vi "ChParamGetRef.vi"(0 "Ch Received in":refnum<vi>, 1 "Channel OFF delay":refnum<vi>, 2 "Channel On Delay in":refnum<vi>, 3 "Number Of Retry in":refnum<vi>, 4 "SW Retry Delay":refnum<vi>, 5 "Retry Delay in":refnum<vi>, 6 "Active on startup":refnum<vi>, 7 "SW Number Of Retry":refnum<vi>, 8 "Reset Status Delay":refnum<vi>, 9 "I/O control":refnum<vi>, 10 "Init":bool, 11 "Current Threshold in":refnum<vi>, 12 "Ch General data":refnum<vi>, 13 "Comm. control":refnum<vi>) -> (14 "Reset Status Delay out":refnum<vi>, 16 "Channel On Delay out":refnum<vi>, 17 "Ch General data out":refnum<vi>, 18 "Channel OFF delay out":refnum<vi>, 19 "Comm. control out":refnum<vi>, 20 "Ch Received out":refnum<vi>, 21 "SW Retry Delay out":refnum<vi>, 22 "Current Threshold  out":refnum<vi>, 23 "Active on startup out":refnum<vi>, 24 "SW Number Of Retry out":refnum<vi>, 25 "Retry Delay out":refnum<vi>, 26 "Number Of Retry out":refnum<vi>, 27 "I/O control out":refnum<vi>)   [LabVIEW 2017]
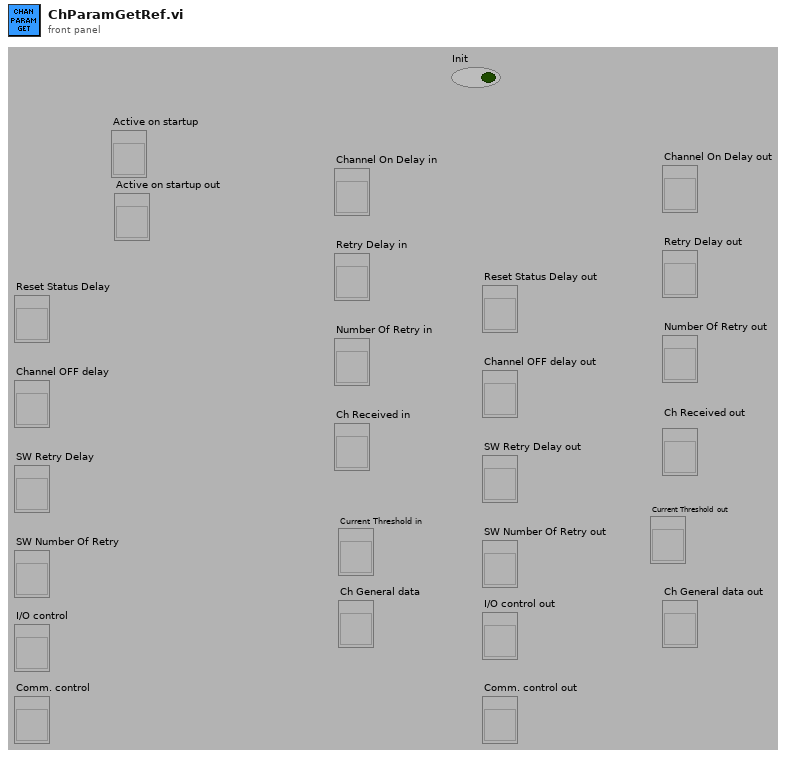
[diagram p1: front panel]
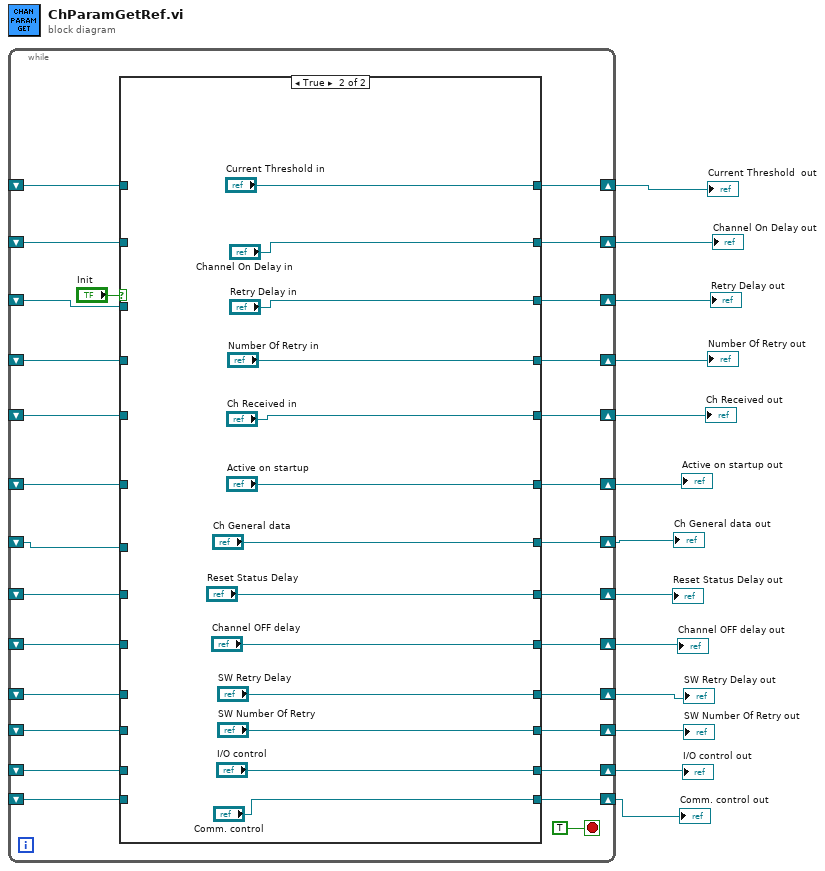
[diagram p0: block diagram]
diagram:
  n1 = while {
    shift-right: [w30] -> w9
    shift-left: _ -> [w36]
    shift-right: [w40] -> w13
    shift-left: _ -> [w35]
    shift-right: [w39] -> w12
    shift-left: _ -> [w34]
    shift-right: [w38] -> w11
    shift-left: _ -> [w33]
    shift-right: [w37] -> w10
    shift-left: _ -> [w32]
    shift-right: [w29] -> w8
    shift-left: _ -> [w28]
    shift-right: [w27] -> w7
    shift-left: _ -> [w26]
    shift-right: [w25] -> w5
    shift-left: _ -> [w19]
    shift-right: [w24] -> w6
    shift-left: _ -> [w18]
    shift-right: [w23] -> w4
    shift-left: _ -> [w17]
    shift-right: [w22] -> w3
    shift-left: _ -> [w16]
    shift-right: [w21] -> w2
    shift-left: _ -> [w15]
    shift-right: [w20] -> w1
    shift-left: _ -> [w14]
    stop <- TRUE stop-if-true
    n2 = case shown="True" "Init" {
      tunnel: [w50 "Current Threshold in"] -> w30
      tunnel: [w54 "Channel On Delay in"] -> w40
      tunnel: [w53 "Retry Delay in"] -> w39
      tunnel: [w52 "Number Of Retry in"] -> w38
      tunnel: [w51 "Ch Received in"] -> w37
      tunnel: w36 -> [w50 _]
      tunnel: w35 -> [w54 _]
      tunnel: w34 -> [w53 _]
      tunnel: w33 -> [w52 _]
      tunnel: w32 -> [w51 _]
      tunnel: [w49 "Active on startup"] -> w29
      tunnel: w28 -> [w49 _]
      tunnel: [w48 "Ch General data"] -> w27
      tunnel: w26 -> [w48 _]
      tunnel: [w47 "Reset Status Delay"] -> w25
      tunnel: [w46 "Channel OFF delay"] -> w24
      tunnel: [w45 "SW Retry Delay"] -> w23
      tunnel: [w44 "SW Number Of Retry"] -> w22
      tunnel: [w43 "I/O control"] -> w21
      tunnel: [w42 "Comm. control"] -> w20
      tunnel: w19 -> [w47 _]
      tunnel: w18 -> [w46 _]
      tunnel: w17 -> [w45 _]
      tunnel: w16 -> [w44 _]
      tunnel: w15 -> [w43 _]
      tunnel: w14 -> [w42 _]
      frame False {
      }
      frame True {
      }
    }
  }
  "Retry Delay out" <- w12
  "Number Of Retry out" <- w11
  "Ch Received out" <- w10
  "Channel On Delay out" <- w13
  "Current Threshold  out" <- w9
  "Active on startup out" <- w8
  "Ch General data out" <- w7
  "SW Retry Delay out" <- w4
  "SW Number Of Retry out" <- w3
  "I/O control out" <- w2
  "Comm. control out" <- w1
  "Reset Status Delay out" <- w5
  "Channel OFF delay out" <- w6
